vi "PH_ImageCalibrator.get Text for Start Procedure Dialog.vi"(0 "i ref in":refnum<vi>, 5 "error in (no error)":errorcluster) -> (14 "i ref out":refnum<vi>, 17 "Dialog Start Procedure":string, 19 "error out":errorcluster)   [LabVIEW 2014, in "PH_ImageCalibrator.lvlib"]
doc: "This VI creates the text for the Start procedure case. The camera is asked for its attributes (which are displayed) and its serial number. The attributes and the serial number are also written to own attributes."
uses:
  PH_ImageCalibrator.lvlib
  PH_Basics/PH_Img_BaseClass/PH_Img_BaseClass.lvlib
  PH_Basics/PH_Cam_BaseClass/PH_Cam_BaseClass.lvlib
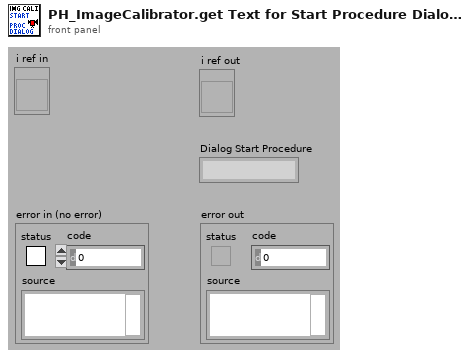
[diagram p1: front panel]
types:
  T1 = cluster{"Cam ID":string, "Gain":dbl, "Brightness":dbl, "Shutter":dbl, "Cam Error":bool, "Mode":i32}
  T2 = typedef "PH_Img_BaseClass.lvlib/PH_Img_BaseClass.i attribute.ctl" = cluster{"GUI Refs":T3, "Timeout Image [ms]":i32, "Default Periodic Period [ms]":i32, "Camera":cluster{"Instancename":string, "Notifier":refnum<notifier>}, "Palette":T4, "Cam Settings":cluster{"Cam ID":string, "Gain":dbl, "Brightness":dbl, "Shutter":dbl, "Cam Info Failure":bool, "Mode":i32}}
  T3 = typedef "PH_Img_BaseClass.lvlib/PH_Img_BaseClass.GUI Refs.ctl" = cluster{"Timeout":refnum<vi>, "Image":refnum<vi>, "Palette":refnum<vi>, "Timeout Set":refnum<vi>}
  T4 = typedef "PH_Img_BaseClass.lvlib/PH_Img_BaseClass.Palette.ctl" = i32
  T5 = typedef "PH_Cam_BaseClass.lvlib/PH_Cam_BaseClass.Settings.ctl" = cluster{"Cam ID":string, "Gain":dbl, "Brightness":dbl, "Shutter":dbl, "Mode":i32}
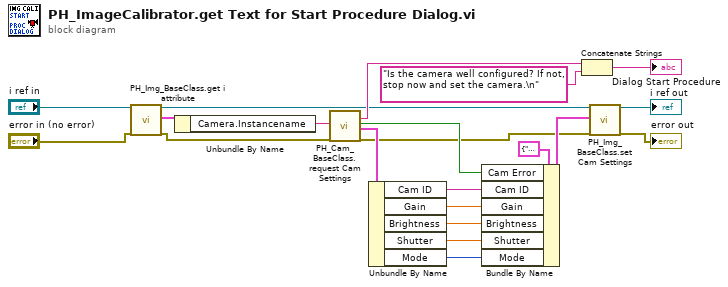
[diagram p0: block diagram]
diagram:
  n1 = call "PH_Img_BaseClass.get i attribute.vi"("i ref in"="i ref in", "error in (no error)"="error in (no error)") -> ("i ref out"=w3:refnum<vi>, "i attribute"=w17:T2, "error out"=w5:errorcluster)  [unwired: 15 in]
  n2 = Unbundle By Name(w17) -> ("Camera.Instancename"=w14:string)
  n3 = call "PH_Cam_BaseClass.request Cam Settings.vi"("Cam Instance"=w14, "error in (no error)"=w5) -> ("Cam Setting Information"=w6:string, "Error getting the Data?"=w13:bool, "Cam Settings"=w7:T5, "error out"=w2:errorcluster)  [unwired: 14 in]
  n4 = Unbundle By Name(w7) -> ("Cam ID"=w12:string, "Gain"=w11:dbl, "Brightness"=w10:dbl, "Shutter"=w9:dbl, "Mode"=w8:i32)
  n5 = Bundle By Name(cluster=T1 {"Cam ID"="", "Gain"=0.0, "Brightness"=0.0, "Shutter"=0.0, "Cam Error"=FALSE, "Mode"=0} ("Cam Settings"), "Cam Error"=w13, "Cam ID"=w12, "Gain"=w11, "Brightness"=w10, "Shutter"=w9, "Mode"=w8) -> (w4:T1)
  n6 = Concatenate Strings(w6, "Is the camera well configured? If not, stop now and set the camera.\n") -> (→"Dialog Start Procedure":string)
  n7 = call "PH_Img_BaseClass.set Cam Settings.vi"("i ref in"=w3, "Cam Settings"=w4, "error in (no error)"=w2) -> ("i ref out"=→"i ref out":refnum<vi>, "error out"=→"error out":errorcluster)  [unwired: 15 in]
